vi "Get Key.vi"(8 "error in":errorcluster, 10 "Sorted Data in":T2, 11 "Refnum in":T1) -> (0 "error out":errorcluster, 1 "Cancel?":bool, 2 "Sorted Data out":T2, 3 "Refnum out":T1)   [LabVIEW 2013]
uses:
  <vilib>/Utility/config.llb/Config Data RefNum.ctl
  <vilib>/Utility/config.llb/Write Key (String).vi
  <vilib>/Utility/config.llb/NI_LVConfig.lvlib
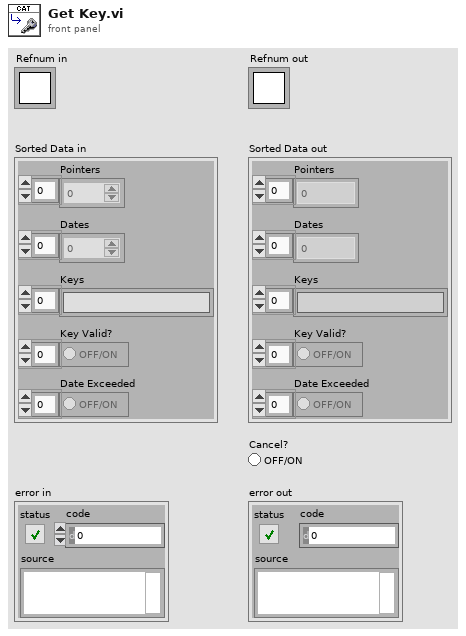
[diagram p1: front panel]
types:
  T1 = typedef "NI_LVConfig.lvlib/Config Data RefNum.ctl" = refnum<k1>
  T2 = cluster{"Pointers":i32[], "Dates":dbl[], "Keys":string[], "Key Valid?":bool[], "Date Exceeded":bool[]}
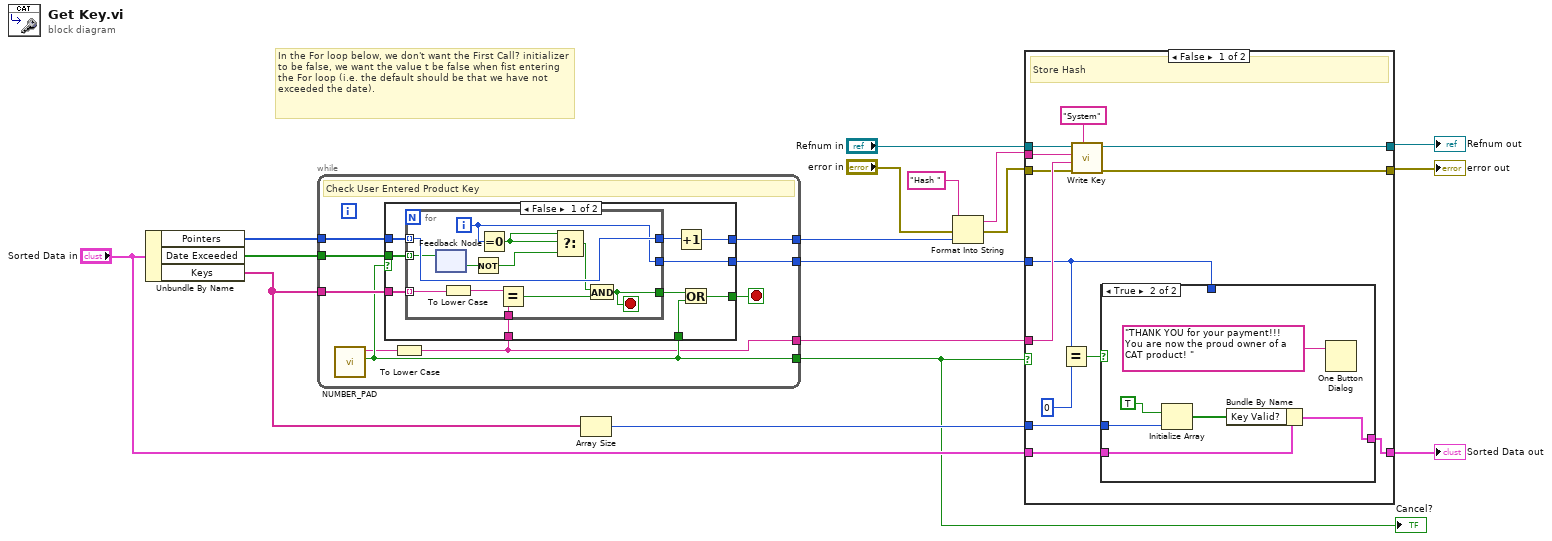
[diagram p0: block diagram]
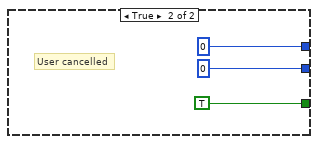
[diagram p2: hidden frame]
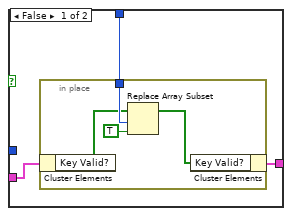
[diagram p3: hidden frame]
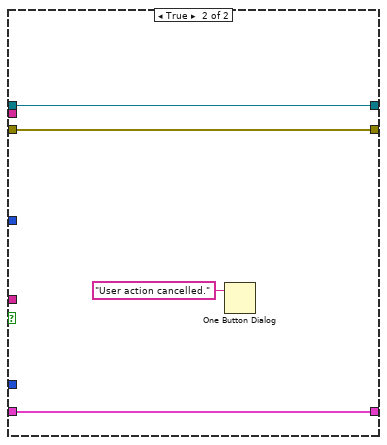
[diagram p4: hidden frame]
diagram:
  # "In the For loop below, we don't want the First Call? initializer to be false, we want the value t be false when fist entering the For loop (i.e. the default should be that we have not exceeded the date)."
  n1 = Unbundle By Name("Sorted Data in") -> ("Pointers"=w10:i32[], "Date Exceeded"=w11:bool[], "Keys"=w15:string[])
  n2 = while {
    tunnel: [w20] -> w7
    tunnel: w15 -> [w25]
    tunnel: [w24] -> w12
    tunnel: [w18] -> w4
    tunnel: w10 -> [w23]
    tunnel: w11 -> [w22]
    tunnel: [w21] -> w13
    stop <- w26 stop-if-true
    # "Check User Entered Product Key"
    n3 = call "NUMBER_PAD.vi"() -> ("Cancel?"=w20:bool, "number (out)"=w19:string)  [unwired: 10 in]
    n4 = To Lower Case(string=w19) -> (all lower case string=w18:string)
    n5 = case shown="False" w20 {
      tunnel: [w36 TRUE] -> w26
      tunnel: w25 -> [w35 _]
      tunnel: [w32 0] -> w24
      tunnel: w18 -> [w31 _]
      tunnel: w20 -> [w30 _]
      tunnel: w23 -> [w29 _]
      tunnel: w22 -> [w28 _]
      tunnel: [w27 0] -> w21
      frame False {
        n6 = for {
          tunnel: w35 -> [w38] mode=indexing
          tunnel: w31 -> [w48]
          tunnel: [w46] -> w34
          tunnel: [w45] -> w33
          tunnel: w29 -> [w45] mode=indexing
          tunnel: w28 -> [w44] mode=indexing
          tunnel: [w42] -> w27
          i -> [w42]
          stop <- w46 stop-if-true
          n7 = feedback-in #1(w44) -> ()
          n8 = feedback #1() -> (w43:bool)  [unwired: 1 in]
          n9 = To Lower Case(string=w38) -> (all lower case string=w37:string)
          n10 = Not(x=w43) -> (.not. x?=w40:bool)
          n11 = Equal To 0?(x=w42) -> (x = 0?=w41:bool)
          n12 = Equal?(x=w37, y=w48) -> (x = y?=w47:bool)
          n13 = Select(t=w41, s=w41, f=w40) -> (s? t:f=w39:bool)
          n14 = And(x=w39, y=w47) -> (x .and. y?=w46:bool)
        }
        n15 = Increment(x=w33) -> (x+1=w32:i32)
        n16 = Or(x=w34, y=w30) -> (x .or. y?=w36:bool)
      }
      frame True {
        # "User cancelled"
      }
    }
  }
  "Cancel?" <- w7
  n17 = Array Size(array=w15) -> (size(s)=w16:i32)
  n18 = Format Into String(initial string="Hash " ("key"), error in="error in", w12) -> (resulting string=w5:string, error out=w6:errorcluster)  [unwired: 1 in]
  n19 = case shown="False" w7 {
    tunnel: "Refnum in" -> [w64 w81]
    tunnel: [w63 w81] -> w8
    tunnel: [w62 w80] -> w9
    tunnel: w4 -> [w60 _]
    tunnel: w5 -> [w59 _]
    tunnel: w6 -> [w58 w80]
    tunnel: w13 -> [w53 _]
    tunnel: "Sorted Data in" -> [w55 w79]
    tunnel: w16 -> [w54 _]
    tunnel: [w52 w79] -> w17
    frame False {
      # "Store Hash"
      n20 = Equal?(x=w53, y=0) -> (x = y?=w56:bool)
      n21 = call-poly <vilib>:"Write Key.vi"("section"="System", "error in (no error)"=w58, "value"=w60, "key"=w59, "refnum"=w64) -> ("error out"=w62:errorcluster, "refnum out"=w63:T1)  [unwired: 4 in, 1 out]
      n22 = case shown="True" w56 {
        tunnel: w55 -> [w67 w76]
        tunnel: w54 -> [_ w74]
        tunnel: w53 -> [w66 _]
        tunnel: [w65 w72] -> w52
        frame False {
          n23 = in-place {
            in-place-border: w66 -> [w71]
            n24 = in-place-cluster #2(w67) -> ("Key Valid?"=w70:bool[])
            n25 = Replace Array Subset(array=w70, new element=TRUE ("new element/subarray"), index=w71) -> (w68:bool[])
            n26 = in-place-cluster #2("Key Valid?"=w68) -> (w65:T2)
          }
        }
        frame True {
          n27 = Initialize Array(TRUE, w74) -> (w73:bool[])
          n28 = Bundle By Name(cluster=w76, "Key Valid?"=w73) -> (w72:T2)
          n29 = One Button Dialog(message="THANK YOU for your payment!!!  You are now the proud owner of a CAT product! ") -> ()  [unwired: 1 in, 1 out]
        }
      }
    }
    frame True {
      n30 = One Button Dialog(message="User action cancelled.") -> ()  [unwired: 1 in, 1 out]
    }
  }
  "Sorted Data out" <- w17
  "error out" <- w9
  "Refnum out" <- w8
